vi "Fetch Task from Map.vi"(0 "Task map in":map{string, refnum<k21>}(c390), 5 "Task in":refnum<k21>, 11 "error in (no error)":errorcluster) -> (4 "Task out":refnum<k21>, 6 "Session Name":string, 15 "error out":errorcluster)   [LabVIEW 2021, in "NI DAQmx_wrapper.lvlib"]
uses:
  NI DAQmx_wrapper.lvlib
  <vilib>/Utility/error.llb/Error Cluster From Error Code.vi
  <vilib>/ErrorRing/Error Ring.xnode
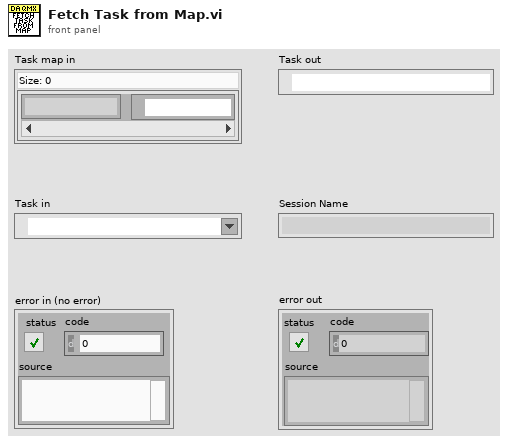
[diagram p1: front panel]
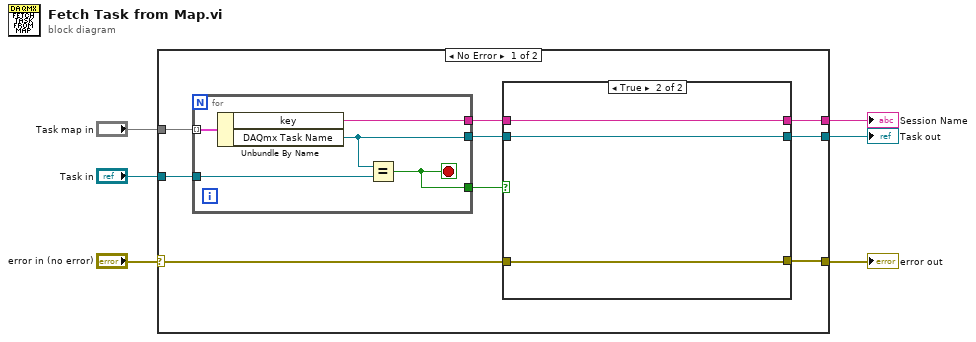
[diagram p0: block diagram]
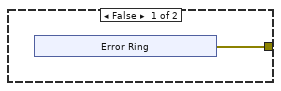
[diagram p2: hidden frame]
diagram:
  n1 = case shown="No Error" "error in (no error)" {
    selector: "error in (no error)" -> [w11 w30]
    tunnel: "Task map in" -> [w15 _]
    tunnel: [w9 _] -> w4
    tunnel: [w10 w30] -> w3
    tunnel: "Task in" -> [w14 _]
    tunnel: [w7 _] -> w1
    frame No Error {
      n2 = for {
        tunnel: w15 -> [w29] mode=indexing
        tunnel: w14 -> [w28]
        tunnel: [w27] -> w12
        tunnel: [w26] -> w13
        tunnel: [w25] -> w8
        stop <- w26 stop-if-true
        n3 = Unbundle By Name(w29) -> ("key"=w25:string, "DAQmx Task Name"=w27:refnum<k21>)
        n4 = Equal?(x=w27, y=w28) -> (x = y?=w26:bool)
      }
      n5 = case shown="True" w13 {
        tunnel: w12 -> [_ w23]
        tunnel: w11 -> [_ w24]
        tunnel: [w16 w24] -> w10
        tunnel: [_ w23] -> w9
        tunnel: w8 -> [_ w22]
        tunnel: [_ w22] -> w7
        frame False {
          n6 = xnode "Error Ring"() -> ("error out"=w16:errorcluster)
        }
        frame True {
        }
      }
    }
    frame Error {
    }
  }
  "Task out" <- w4
  "error out" <- w3
  "Session Name" <- w1
